vi "LINX - Blink_mod_Trig_sendot_prot_new changes.vi"(10 "Data pipeline  python file (hist_calc.py)":path=path "C:/Users/TIDAS/OneDrive - University of Gothenburg/TietzeLab/Autodata_Exp/Pyhton scripts_labview/Script for Stage II_labview/Save_data.py", 11 "File save\\ operating folder":path=path "C:/Users/TIDAS/OneDrive - University of Gothenburg/TietzeLab/Autodata_Exp/21112022_Con_selfetch_func_XXMumSE15_HS_5conc_sen&sel0.5V20points") -> ()   [LabVIEW 2021]
doc: "Manually blink and LED attached to a digital output channel of a LINX device by clicking and LED control in LabVIEW."
uses:
  <vilib>/MakerHub/LINX/Public/Peripherals/Digital/Digital Read 1 Chan.vi
  <vilib>/MakerHub/LINX/Public/Peripherals/Digital/Digital Write 1 Chan.vi
  <vilib>/MakerHub/LINX/Public/Peripherals/Digital/Digital Read N Chans.vi
  <vilib>/MakerHub/LINX/Public/Peripherals/Digital/Digital Write N Chans.vi
  <vilib>/MakerHub/LINX/Private/Local IO/LinxDigitalRead.vi
  <vilib>/MakerHub/LINX/Public/Utilities/Check Channel.vi
  <vilib>/MakerHub/LINX/Private/Local IO/LinxDigitalWrite.vi
  <vilib>/MakerHub/LINX/Public/Utilities/Open Serial.vi
  <vilib>/MakerHub/LINX/Private/Utilties/Generate Error.vi
  <vilib>/MakerHub/LINX/LMH-LINX.lvlib
panel:
  in  "milliseconds to wait between readings":u32=9000
  in  "DO Channel":u8=8
  out "I-V-Wash":cluster{dbl[], dbl[]}(graph)
  out "Current - wash":cluster{dbl[], dbl[]}(graph)
  out "Voltage -Wash":cluster{dbl[], dbl[]}(graph)
  out "Amplitude vs TimeStamp 2":cluster{dbl[], dbl[]}(graph)
  out "CTC PAL wash Iteration":dbl
  in  "Arduino pin for \nPhase 1\nTrigger calculation":u8=7
  out "CTC PAL conc Iteration":dbl
  in  "Intitializer Value":dbl
  in  "Conc cases start\n@ 0":dbl=8.0 format="%#_13g"
  in  "Baud Rate Override":u32=9600
  out "Amplitude vs TimeStamp-sample":cluster{dbl[], dbl[]}(graph)
  in  "No. of Reading":i32=3
  in  "Sendot port":refnum<visa-resource-name>="COM3"
  in  "DI Channel-Wash":u8=4
  in  "VISA resource name 2":refnum<visa-resource-name>="COM4"
  in  "Waveform":i16(ring)=2 items=["Sin", "Cos", "Triang", "Square", "Saw Tooth", "Inc Ramp", "Dec Ramp", "White Noise"]
  out "Voltage-sample":cluster{dbl[], dbl[]}(graph)
  out "Current":cluster{dbl[], dbl[]}(graph)
  in  "N points/period":dbl=40.0 format="%#_13g"
  in  "amplitude":dbl=-1.0 format="%#_13g"
  in  "Enable Voltage Source (F: Disable)":bool=TRUE
  in  "dc offset":dbl format="%#_13g"
  in  "N periods":dbl=3.0 format="%#_13g"
  out "I-V":cluster{dbl[], dbl[]}(graph)
  out "Loop Rate (Hz)":u32=12
  out "LED Value":bool
  in  "DI Channel-sample":u8=2
  in  "Serial Port":refnum<visa-resource-name>="COM1"
  in  "Stop Button":bool
  # "LINX Device Settings"
  # "LED Control"
  # "Circuit Schematic"
  # "^^ Click Here ^^"
  # "Manual Blink Example\n\nThis example demonstrates how to blink an LED on a LINX device by clicking on an LED control in LabVIEW.\n\nInstructions\n1. Select the Serial Port associated with the LINX Device.\n2. Select the Digital Output Channel connected to the LED.\n3. Click the Run Arrow."
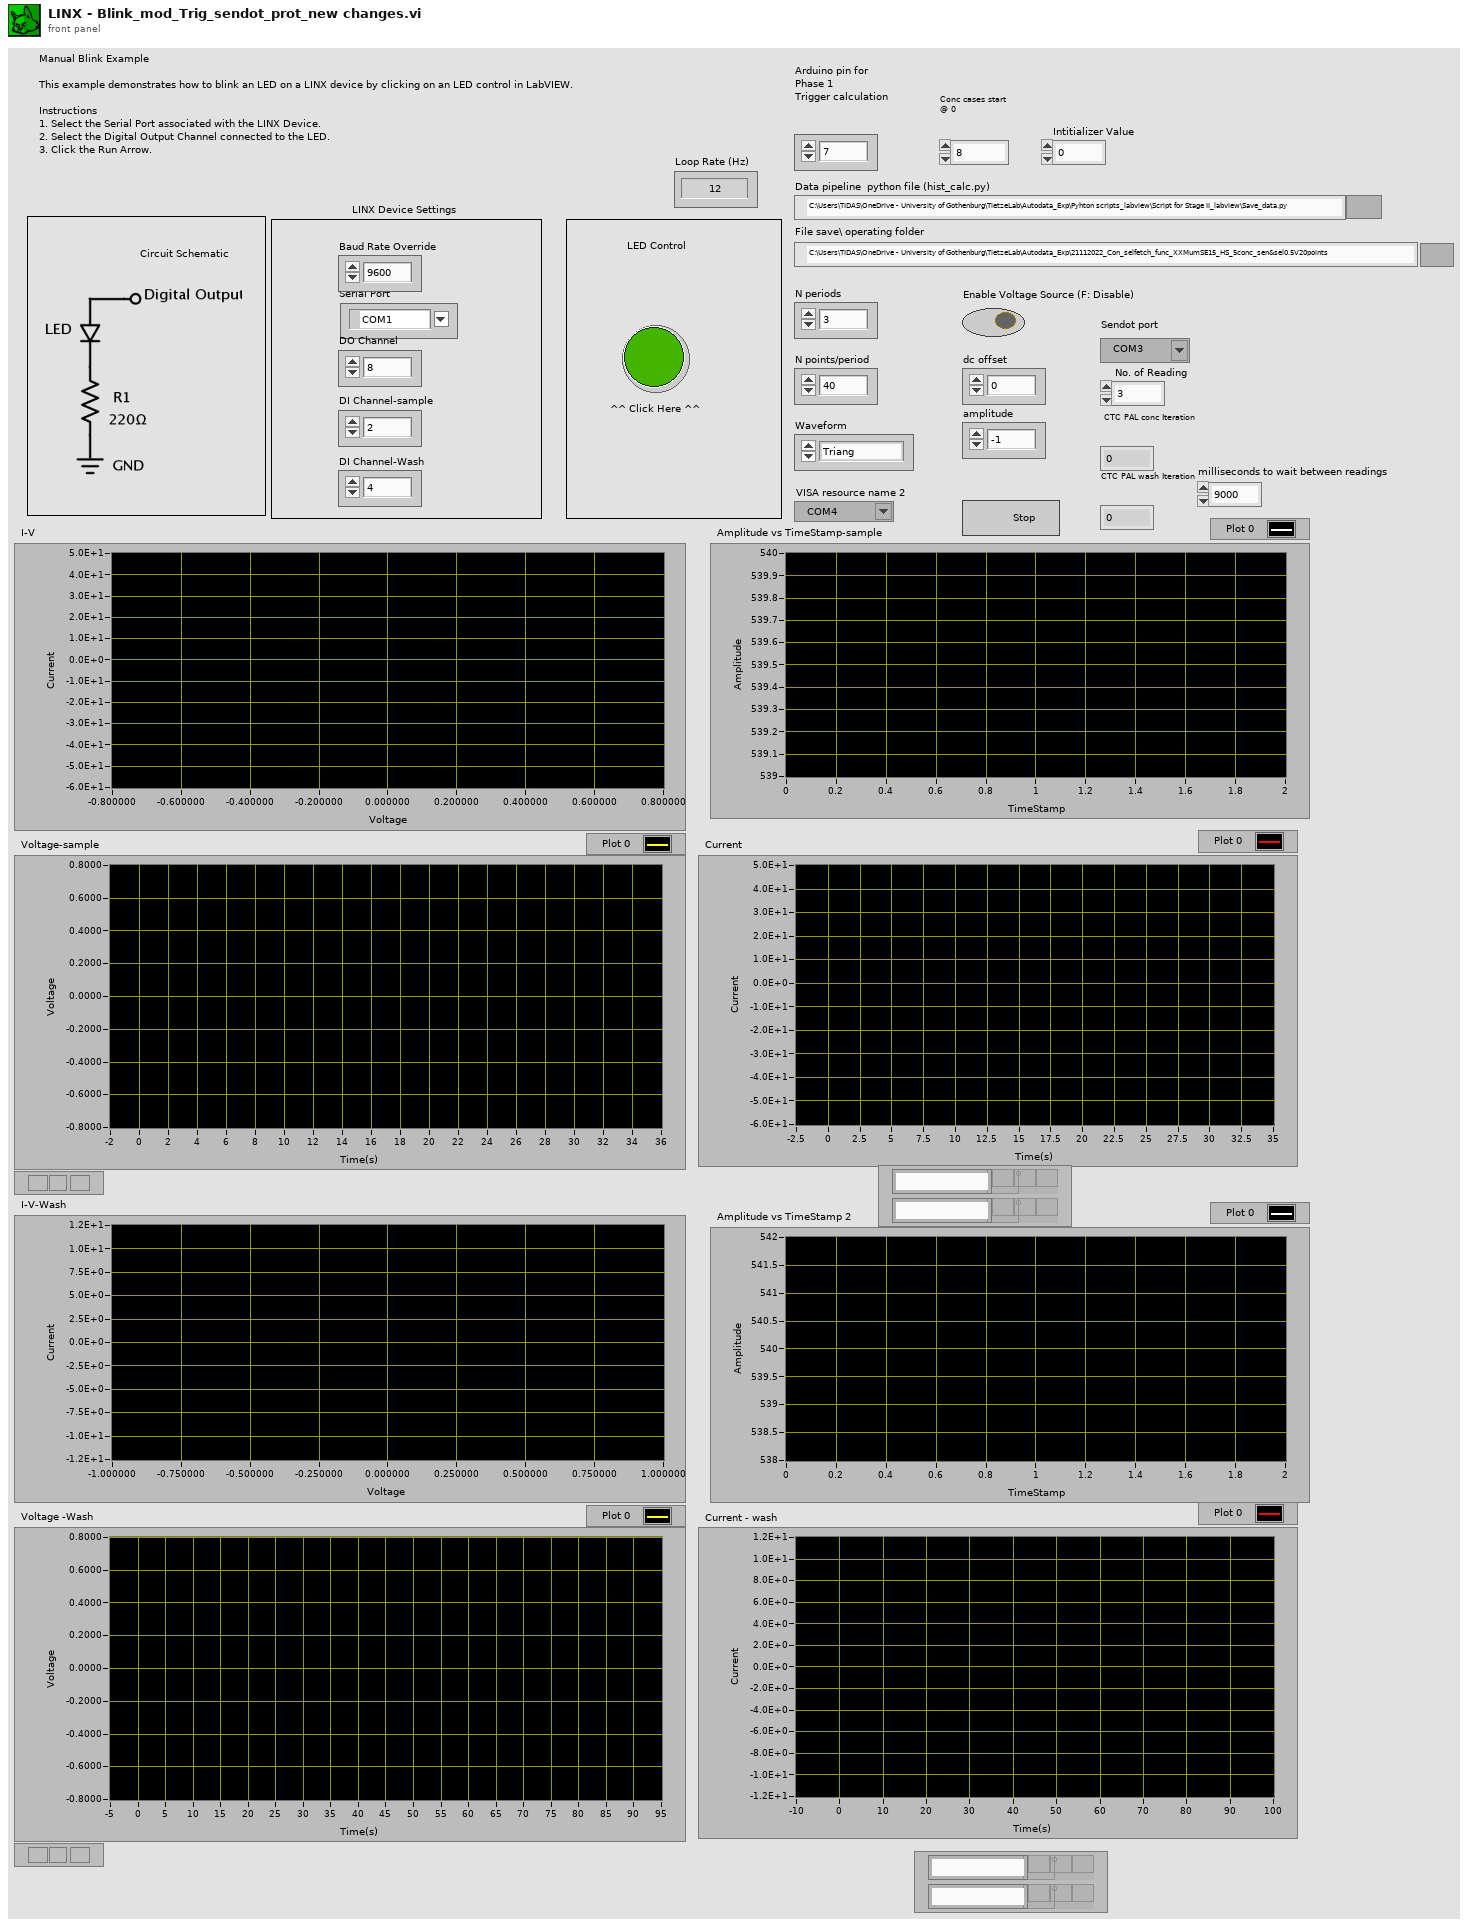
[diagram p1: front panel]
types:
  T1 = typedef "LMH-LINX.lvlib/LINX Ref.ctl" = cluster{"IO":T2, "Interface":T3, "LINX Device Config":T4}
  T2 = typedef "LMH-LINX.lvlib/Platform.ctl" = enum16{"Remote", "Local"}
  T3 = typedef "LMH-LINX.lvlib/Interface.ctl" = enum16{"Serial", "TCP"}
  T4 = typedef "LMH-LINX.lvlib/Device.lvlib/LINX Device Config.ctl" = cluster{"Interface":T3, "COM Port":refnum<visa-resource-name>, "TCP Configuration":T5, "Device Family":u8, "Device ID":u8, "Device Name":string, "TCP Ref":refnum<k5>, "Channels":T6}
  T5 = typedef "LMH-LINX.lvlib/Device.lvlib/TCP Config.ctl" = cluster{"IP Address":string, "Port":u16}
  T6 = typedef "LMH-LINX.lvlib/Channels.ctl" = cluster{"DI":u8[], "DO":u8[], "AI":u8[], "AO":u8[], "PWM":u8[], "QE":u8[], "UART":u8[], "I2C 2":u8[], "SPI":u8[], "CAN":u8[], "Servo":u8[], "AI Ref (V)":dbl, "AI Resolution (Bits)":u8, "AO Ref (V)":dbl, "AO Resolution (Bits)":u8}
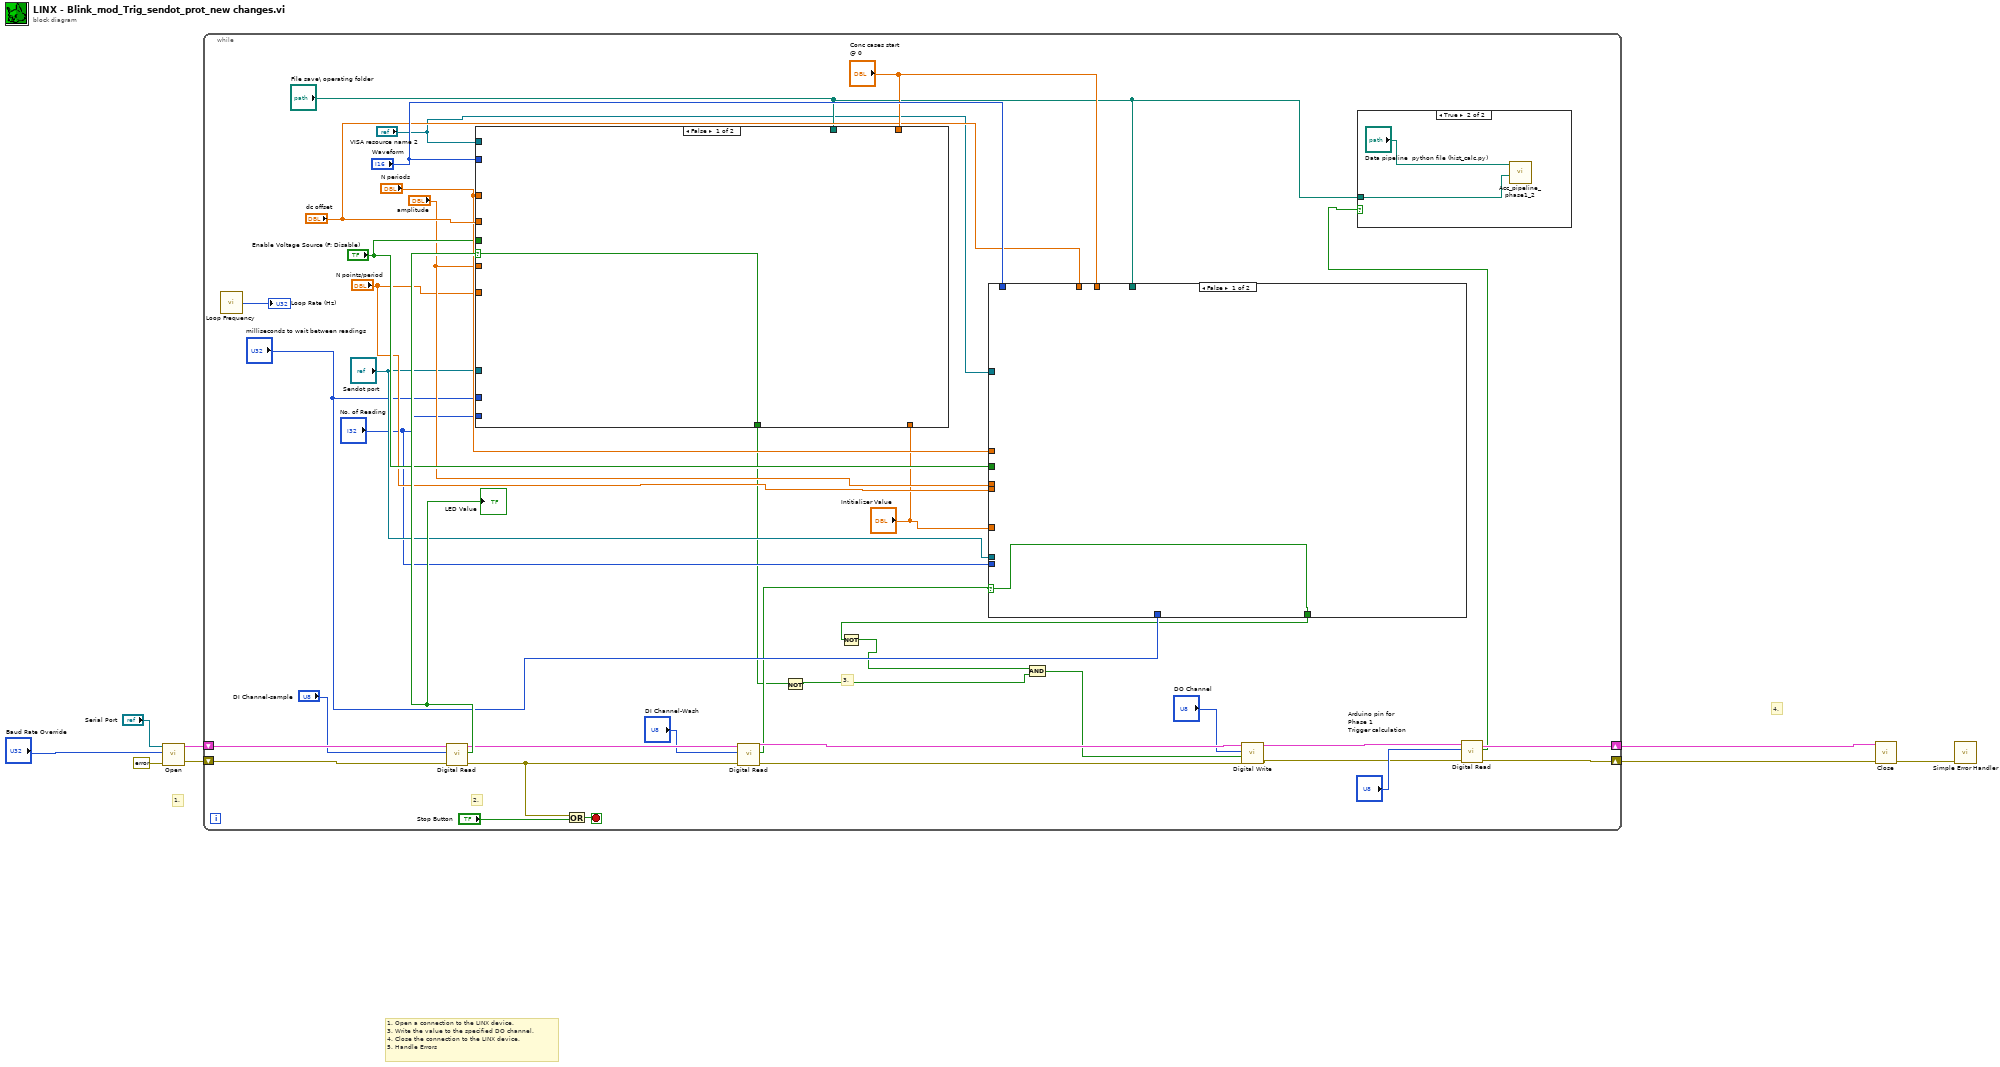
[diagram p0: block diagram]
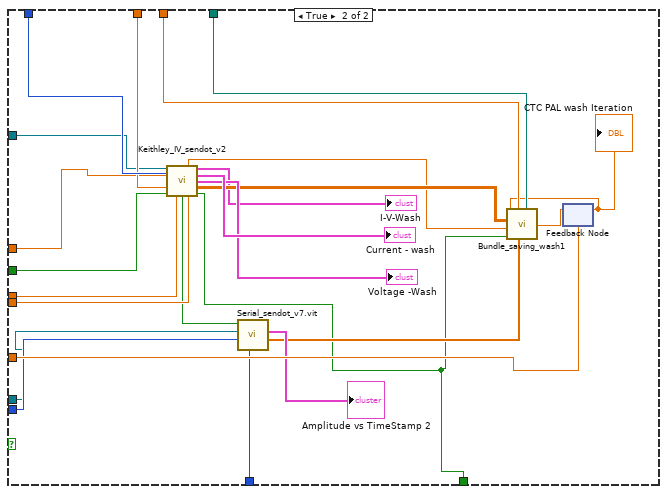
[diagram p3: hidden frame]
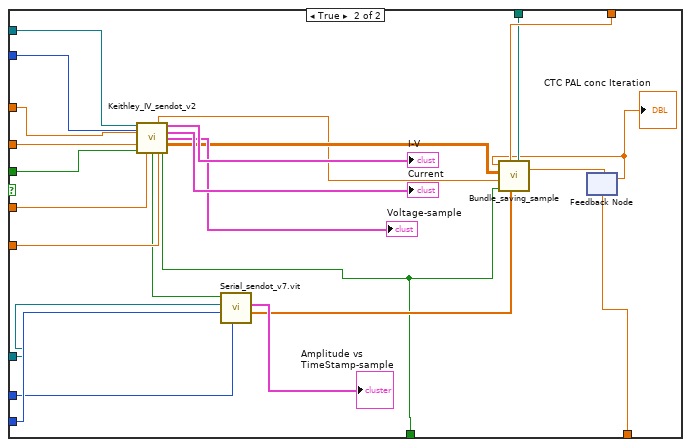
[diagram p4: hidden frame]
diagram:
  # "1. Open a connection to the LINX device.\n3. Write the value to the specified DO channel.\n4. Close the connection to the LINX device.\n5. Handle Errors"
  # "4."
  # "3."
  # "1."
  n1 = call-poly <vilib>:"Open.vi"("Error In"=errorcluster {"status"=FALSE, "code"=0, "source"=""}, "Baud Rate Override"="Baud Rate Override", "Serial Port"="Serial Port") -> ("Error Out"=w7:errorcluster, "LINX Resource"=w8:T1)  [unwired: 6 in, 1 out]
  n2 = while {
    shift-right: [w40] -> w6
    shift-left: w7 -> [w43]
    shift-right: [w38] -> w2
    shift-left: w8 -> [w44]
    stop <- w46 stop-if-true
    # "2."
    n3 = call <vilib>:"Loop Frequency.vi"() -> ("Loop Rate (Hz)"=→"Loop Rate (Hz)":u32)
    n4 = call-poly <vilib>:"Digital Read.vi"("Error In"=w43, "DI Channel"="DI Channel-sample", "LINX Resource"=w44) -> ("Error Out"=w36:errorcluster, "DI Value"=w39:bool, "LINX Resource"=w37:T1)  [unwired: 6 in]
    "LED Value" <- w39
    n5 = case shown="False" w39 {
      selector: w39 -> [w74 _]
      tunnel: "amplitude" -> [_ w95]
      tunnel: "dc offset" -> [_ w94]
      tunnel: "VISA resource name 2" -> [_ w93]
      tunnel: "Conc cases start\n@ 0" -> [_ w87]
      tunnel: "Waveform" -> [_ w92]
      tunnel: "Enable Voltage Source (F: Disable)" -> [_ w91]
      tunnel: "N points/period" -> [_ w90]
      tunnel: "Sendot port" -> [_ w80]
      tunnel: "No. of Reading" -> [_ w81]
      tunnel: "Intitializer Value" -> [_ w89]
      tunnel: "N periods" -> [_ w88]
      tunnel: "File save\\ operating folder" -> [_ w86]
      tunnel: [w74 w75] -> w10
      tunnel: "milliseconds to wait between readings" -> [_ w76]
      frame False {
      }
      frame True {
        n6 = call "Keithley_IV_sendot_v2.vi"("VISA resource name 2"=w93, "Waveform"=w92, "N periods"=w88, "dc offset"=w94, "Enable Voltage Source (F: Disable)"=w91, "amplitude"=w95, "N points/period"=w90) -> ("x*y"=w84:dbl, "I-V"=→"I-V":cluster{dbl[], dbl[]}, "Current"=→"Current":cluster{dbl[], dbl[]}, "Voltage"=→"Voltage-sample":cluster{dbl[], dbl[]}, "Appened output array"=w85:dbl[][], "Bool to sendot savineg"=w77:bool, "x = y?"=w75:bool)  [unwired: 2 in]
        n7 = call "Serial_sendot_v7.vit"("milliseconds to wait between readings"=w76, "Numeric 2"=w81, "VISA resource name"=w80, "Arduino"=w77) -> ("Array"=w78:dbl[], "Amplitude vs TimeStamp"=→"Amplitude vs TimeStamp-sample":cluster{dbl[], dbl[]})  [unwired: 5 in]
        n8 = feedback #1(w89) -> (w82:dbl)
        "CTC PAL conc Iteration" <- w82
        n9 = call "Bundle_saving_sample.vi"("File saving directory/folder"=w86, "new element/subarray"=w78, "Conc cases start @ 0"=w87, "Boolean"=w75, "Numeric"=w84, "Array"=w85, "Intitializer Value"=w82) -> ("Intitializer Value 2"=w83:dbl)  [unwired: 4 in]
        n10 = feedback-in #1(w83) -> ()
      }
    }
    n11 = Or(x=w36, y="Stop Button") -> (x .or. y?=w46:bool)
    n12 = call-poly <vilib>:"Digital Read.vi"("Error In"=w36, "DI Channel"="DI Channel-Wash", "LINX Resource"=w37) -> ("Error Out"=w19:errorcluster, "DI Value"=w13:bool, "LINX Resource"=w21:T1)  [unwired: 6 in]
    n13 = Not(x=w10) -> (.not. x?=w9:bool)
    n14 = case shown="False" w13 {
      selector: w13 -> [w49 _]
      tunnel: "Waveform" -> [_ w73]
      tunnel: "Conc cases start\n@ 0" -> [_ w72]
      tunnel: "dc offset" -> [_ w71]
      tunnel: "N periods" -> [_ w70]
      tunnel: "Enable Voltage Source (F: Disable)" -> [_ w69]
      tunnel: "amplitude" -> [_ w68]
      tunnel: "N points/period" -> [_ w67]
      tunnel: "Intitializer Value" -> [_ w66]
      tunnel: "Sendot port" -> [_ w55]
      tunnel: "No. of Reading" -> [_ w56]
      tunnel: "File save\\ operating folder" -> [_ w65]
      tunnel: "VISA resource name 2" -> [_ w64]
      tunnel: [w49 w50] -> w12
      tunnel: "milliseconds to wait between readings" -> [_ w51]
      frame False {
      }
      frame True {
        n15 = call "Keithley_IV_sendot_v2.vi"("VISA resource name 2"=w64, "Waveform"=w73, "N periods"=w70, "dc offset"=w71, "Enable Voltage Source (F: Disable)"=w69, "amplitude"=w68, "N points/period"=w67) -> ("x*y"=w58:dbl, "I-V"=→"I-V-Wash":cluster{dbl[], dbl[]}, "Current"=→"Current - wash":cluster{dbl[], dbl[]}, "Voltage"=→"Voltage -Wash":cluster{dbl[], dbl[]}, "Appened output array"=w59:dbl[][], "Bool to sendot savineg"=w52:bool, "x = y?"=w50:bool)  [unwired: 2 in]
        n16 = call "Serial_sendot_v7.vit"("milliseconds to wait between readings"=w51, "Numeric 2"=w56, "VISA resource name"=w55, "Arduino"=w52) -> ("Array"=w53:dbl[], "Amplitude vs TimeStamp"=→"Amplitude vs TimeStamp 2":cluster{dbl[], dbl[]})  [unwired: 5 in]
        n17 = feedback #2(w66) -> (w60:dbl)
        "CTC PAL wash Iteration" <- w60
        n18 = call "Bundle_saving_wash1.vi"("File saving directory/folder"=w65, "new element/subarray"=w53, "Conc cases start @ 0"=w72, "Boolean"=w50, "Numeric"=w58, "Array"=w59, "Intitializer Value"=w60) -> ("Intitializer Value 2"=w61:dbl)  [unwired: 4 in]
        n19 = feedback-in #2(w61) -> ()
      }
    }
    n20 = Not(x=w12) -> (.not. x?=w11:bool)
    n21 = And(x=w11, y=w9) -> (x .and. y?=w16:bool)
    n22 = call-poly <vilib>:"Digital Write.vi"("Error In"=w19, "Output Value"=w16, "DO Channel"="DO Channel", "LINX Resource"=w21) -> ("Error Out"=w18:errorcluster, "LINX Resource"=w20:T1)  [unwired: 6 in]
    n23 = call-poly <vilib>:"Digital Read.vi"("Error In"=w18, "DI Channel"="Arduino pin for \nPhase 1\nTrigger calculation", "LINX Resource"=w20) -> ("Error Out"=w40:errorcluster, "DI Value"=w14:bool, "LINX Resource"=w38:T1)  [unwired: 6 in]
    n24 = case shown="True" w14 {
      tunnel: "File save\\ operating folder" -> [_ w47]
      frame False {
      }
      frame True {
        n25 = call "Acc_pipeline_phase1_2.vi"("path 2"=w47, "module path"="Data pipeline  python file (hist_calc.py)") -> ()  [unwired: 10 in]
      }
    }
  }
  n26 = call <vilib>:"Close.vi"("Error In"=w6, "LINX Resource"=w2) -> ("Error Out"=w4:errorcluster)  [unwired: 9 in]
  n27 = call <vilib>:"Simple Error Handler.vi"("error in (no error)"=w4) -> ()  [unwired: 4 in, 5 out]
